vi "calculateDataPoints.vi"(8 "error in (no error)":errorcluster, 11 "PlayFile in":refnum<class "PlayFile.lvclass">) -> (0 "error out":errorcluster, 1 "Data":T2, 2 "TimeArray":dbl[](array[numeric]), 3 "PlayFile out":refnum<class "PlayFile.lvclass">, 4 "dataType":T1(ring))   [LabVIEW 2011, in "Tools.lvlib" / "Scripting.lvlib" / "PlayFile.lvclass"]
uses:
  PlayFile.lvclass
  DatabaseHelpers/Database Objects/Channel/Channel.lvclass
  ScriptEvent.lvclass
panel:
  out "samples":i32
  out "DataArray":dbl[](array[numeric])
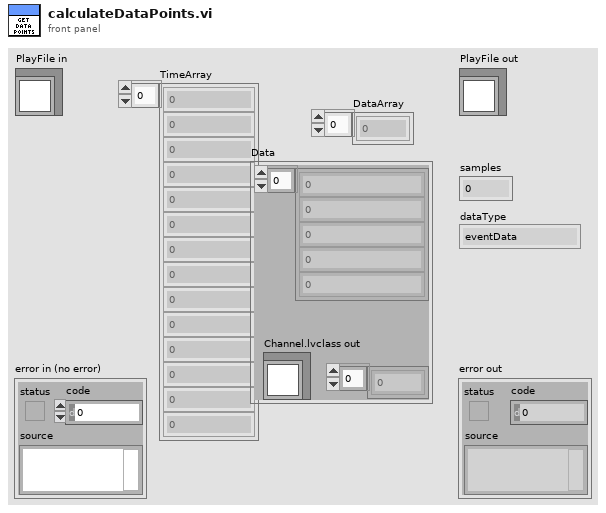
[diagram p1: front panel]
types:
  T1 = enum16{"eventData", "singleToneData", "fileData"}
  T2 = cluster{dbl[], "Channel.lvclass out":refnum<class "Channel.lvclass">, dbl[]}
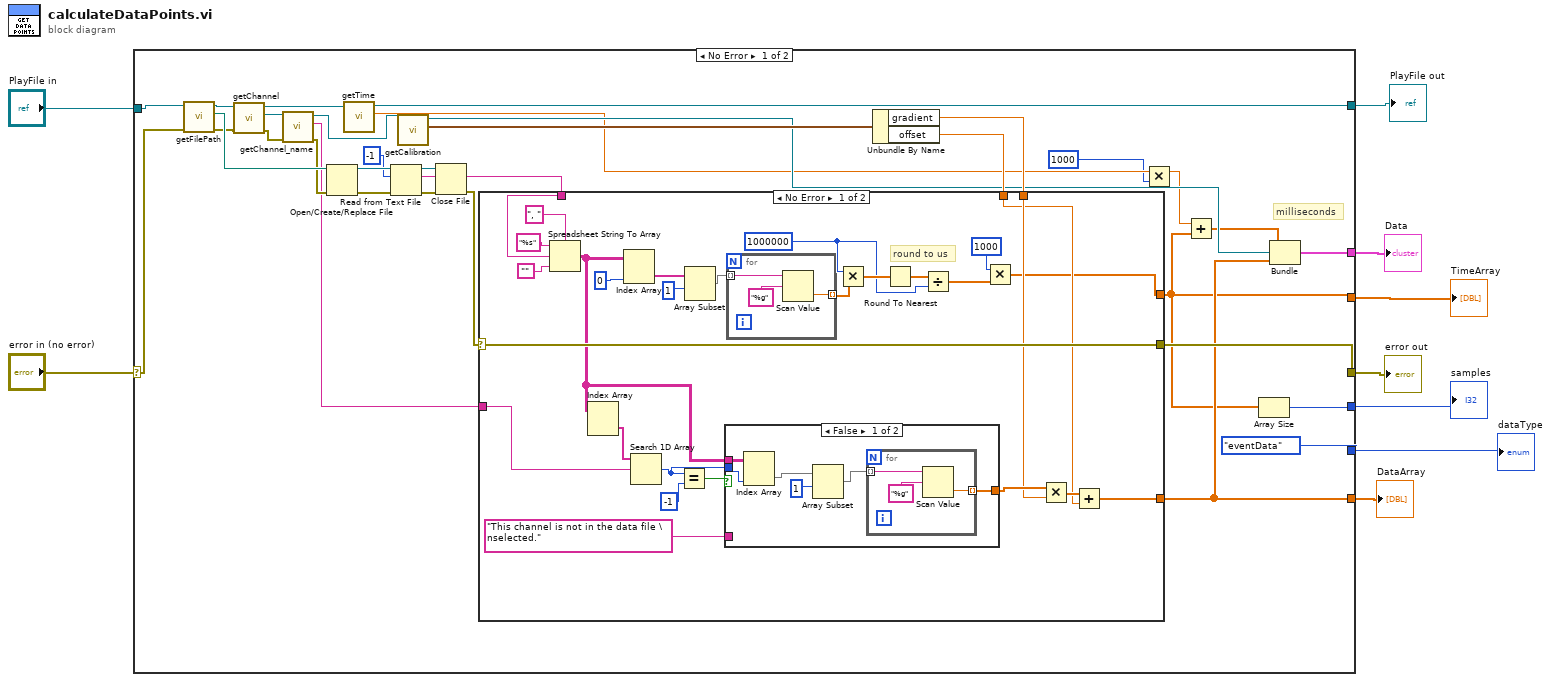
[diagram p0: block diagram]
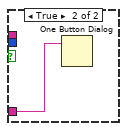
[diagram p2: hidden frame]
diagram:
  n1 = case shown="No Error" "error in (no error)" {
    selector: "error in (no error)" -> [w34 w86]
    tunnel: [w32 w86] -> w8
    tunnel: [w15 w85] -> w6
    tunnel: "PlayFile in" -> [w35 w85]
    tunnel: [w14 _] -> w5
    tunnel: [w20 _] -> w4
    tunnel: [w19 _] -> w3
    tunnel: [w18 _] -> w2
    tunnel: [T1."eventData" ("dataType") _] -> w1
    frame No Error {
      # "milliseconds"
      n2 = call "getFilePath.vi"("error in (no error)"=w34, "PlayFile in"=w35) -> ("error out"=w30:errorcluster, "filePath"=w33:path, "PlayFile out"=w31:refnum<class "PlayFile.lvclass">)  [unwired: 7 in]
      n3 = call-dynamic "getChannel.vi"("error in (no error)"=w30, "ScriptEvent.lvclass in"=w31) -> ("error out"=w28:errorcluster, "Channel.lvclass"=w29:refnum<class "Channel.lvclass">, "ScriptEvent.lvclass out"=w16:refnum<class "PlayFile.lvclass">)  [unwired: 7 in]
      n4 = call "getChannel_name.vi"("error in (no error)"=w28, "Channel.lvclass in"=w29) -> ("error out"=w27:errorcluster, "channel_name"=w26:string, "Channel.lvclass out"=w24:refnum<class "Channel.lvclass">)  [unwired: 7 in]
      n5 = Open/Create/Replace File(file path (use dialog)=w33, error in=w27) -> (refnum out=w42:refnum<file>, error out=w41:errorcluster)  [unwired: 4 in, 1 out]
      n6 = call "getTime.vi"("ScriptEvent.lvclass in"=w16) -> ("time"=w13:dbl, "ScriptEvent.lvclass out"=w15:refnum<class "PlayFile.lvclass">)  [unwired: 8 in, 1 out]
      n7 = Read from Text File(file (use dialog)=w42, count=-1, error in=w41) -> (refnum out=w39:refnum<file>, text=w37:string, error out=w40:errorcluster)  [unwired: 1 in, 1 out]
      n8 = call "getCalibration.vi"("Channel.lvclass in"=w24) -> ("calibration"=w25:cluster{"gradient":dbl, "offset":dbl}, "Channel.lvclass out"=w21:refnum<class "Channel.lvclass">)  [unwired: 8 in, 1 out]
      n9 = Close File(refnum=w39, error in=w40) -> (error out=w36:errorcluster)  [unwired: 1 out]
      n10 = Unbundle By Name(w25) -> ("gradient"=w22:dbl, "offset"=w23:dbl)
      n11 = case shown="No Error" w36 {
        selector: w36 -> [w65 w84]
        tunnel: w37 -> [w70 _]
        tunnel: [w65 w84] -> w32
        tunnel: [w46 _] -> w14
        tunnel: w26 -> [w55 _]
        tunnel: w23 -> [w50 _]
        tunnel: w22 -> [w52 _]
        tunnel: [w49 _] -> w20
        frame No Error {
          w61 = 1000000
          # "round to us"
          n12 = Spreadsheet String To Array(delimiter (Tab)=", ", format string="%s", spreadsheet string=w70, array type (2D Dbl)="") -> (array=w54:string[][])
          n13 = Index Array(array=w54) -> (element=w60:string[])  [unwired: 2 in]
          n14 = Index Array(array=w54, index (col)=0 ("disabled index (col)")) -> (element=w44:string[])  [unwired: 1 in]
          n15 = Search 1D Array(1D array=w60, element=w55) -> (index of element=w56:i32)  [unwired: 1 in]
          n16 = Equal?(x=w56, y=-1) -> (x = y?=w58:bool)
          n17 = Array Subset(array=w44, index=1) -> (w43:string[])  [unwired: 1 in]
          n18 = case shown="False" w58 {
            tunnel: "This channel is not in the data file \nselected." -> [_ w80]
            tunnel: w54 -> [w75 _]
            tunnel: w56 -> [w74 _]
            tunnel: [w71 _] -> w53
            frame False {
              n19 = Index Array(array=w75, index (col)=w74) -> (element=w76:string[])  [unwired: 1 in]
              n20 = Array Subset(array=w76, index=1) -> (w72:string[])  [unwired: 1 in]
              n21 = for {
                tunnel: w72 -> [w79] mode=indexing
                tunnel: [w77] -> w71 mode=indexing
                n22 = Scan Value(string=w79, format string="%g") -> (value=w77:dbl)  [unwired: 1 in, 1 out]
              }
            }
            frame True {
              n23 = One Button Dialog(message=w80) -> ()  [unwired: 1 in, 1 out]
            }
          }
          n24 = for {
            tunnel: w43 -> [w83] mode=indexing
            tunnel: [w81] -> w62 mode=indexing
            n25 = Scan Value(string=w83, format string="%g") -> (value=w81:dbl)  [unwired: 1 in, 1 out]
          }
          n26 = Multiply(x=w61, y=w62) -> (x*y=w64:dbl[])
          n27 = Round To Nearest(number=w64) -> (nearest integer value=w63:dbl[])
          n28 = Divide(x=w63, y=w61) -> (x/y=w47:dbl[])
          n29 = Multiply(x=1000, y=w47) -> (x*y=w46:dbl[])
          n30 = Multiply(x=w53, y=w52) -> (x*y=w51:dbl[])
          n31 = Add(x=w51, y=w50) -> (x+y=w49:dbl[])
        }
        frame Error {
        }
      }
      n32 = Multiply(x=w13, y=1000) -> (x*y=w11:dbl)
      n33 = Add(x=w11, y=w14) -> (x+y=w12:dbl[])
      n34 = Array Size(array=w14) -> (size(s)=w18:i32)
      n35 = Bundle(w12, "Channel.lvclass out"=w21, w20) -> (w19:T2)  [unwired: 1 in]
    }
    frame Error {
    }
  }
  "error out" <- w8
  "PlayFile out" <- w6
  "TimeArray" <- w5
  "DataArray" <- w4
  "Data" <- w3
  "dataType" <- w1
  "samples" <- w2
